vi "FL_Calculate_phi_theta_etc_for_saving.vi"(3 "Mouse face dir. swap":bool, 4 "Input cluster of data":T1) -> (1 "Output data cluster":T2)   [LabVIEW 2016]
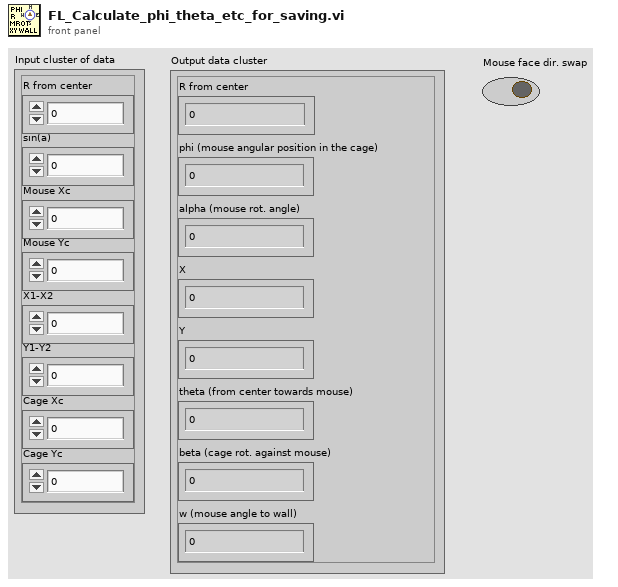
[diagram p1: front panel]
types:
  T1 = cluster{"R from center":dbl, "sin(a)":dbl, "Mouse Xc":dbl, "Mouse Yc":dbl, "X1-X2":dbl, "Y1-Y2":dbl, "Cage Xc":dbl, "Cage Yc":dbl}
  T2 = cluster{"R from center":dbl, "phi (mouse angular position in the cage)":dbl, "alpha (mouse rot. angle)":sgl, "X":dbl, "Y":dbl, "theta (from center towards mouse)":dbl, "beta (cage rot. against mouse)":sgl, "w (mouse angle to wall)":dbl}
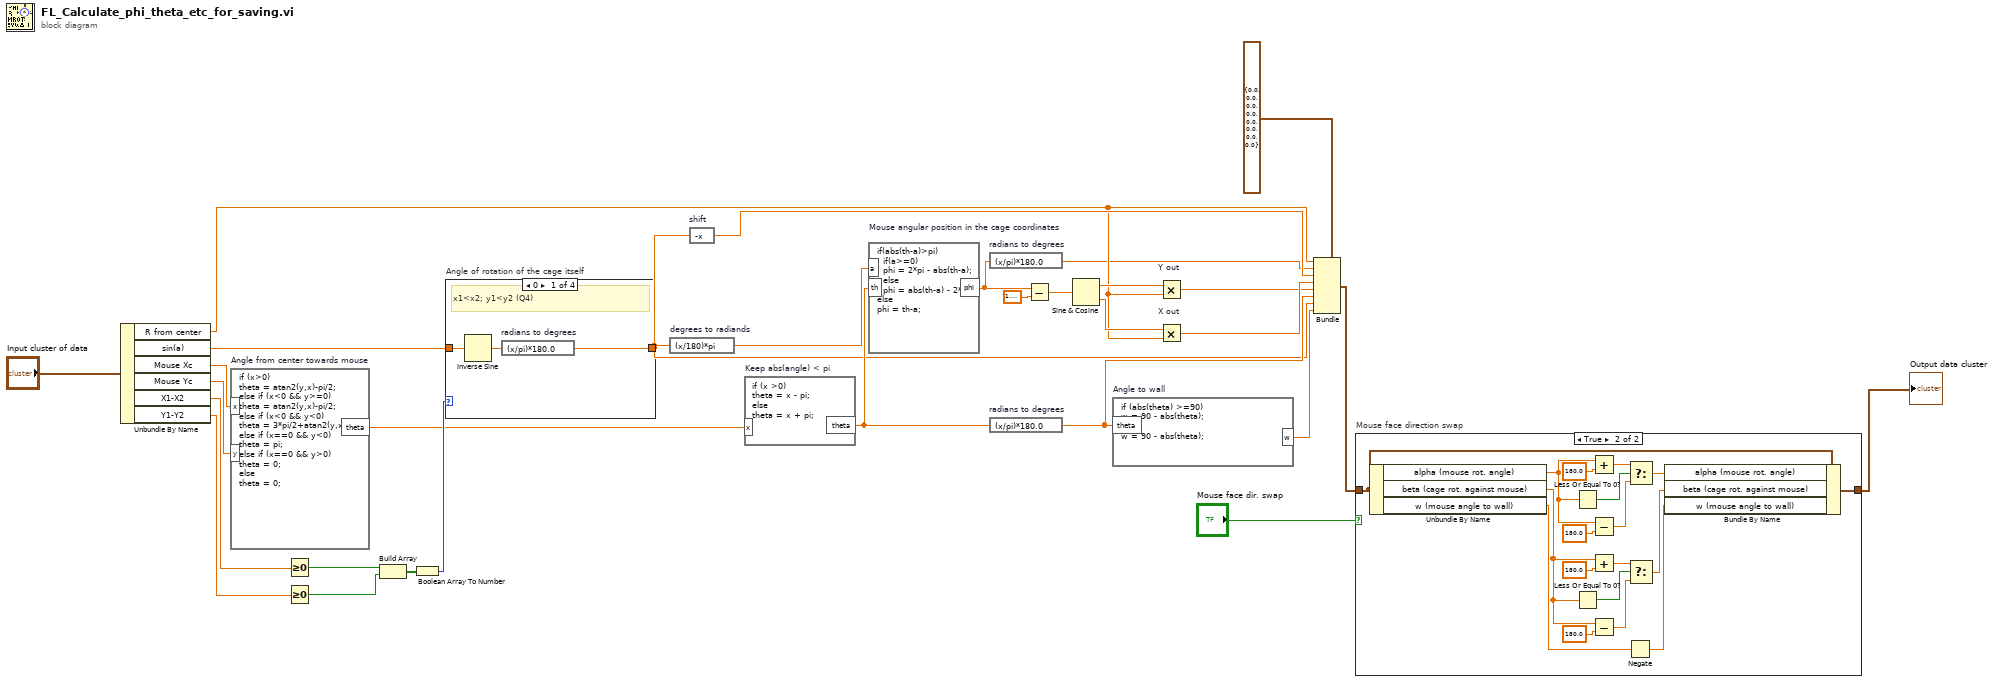
[diagram p0: block diagram]
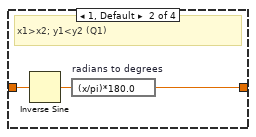
[diagram p3: hidden frame]
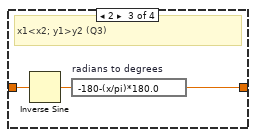
[diagram p4: hidden frame]
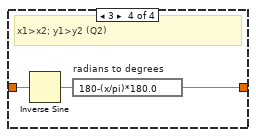
[diagram p5: hidden frame]
diagram:
  n1 = Unbundle By Name("Input cluster of data") -> ("R from center"=w6:dbl, "sin(a)"=w12:dbl, "Mouse Xc"=w11:dbl, "Mouse Yc"=w10:dbl, "X1-X2"=w9:dbl, "Y1-Y2"=w8:dbl)
  n2 = formula code="if (x>0)\ntheta = atan2(y,x)-pi/2;\nelse if (x<0 && y>=0)\ntheta = atan2(y,x)-pi/2;\nelse if (x<0 && y<0)\ntheta = 3*pi/2+atan2(y,x);\nelse if (x==0 && y<0)\ntheta = pi;\nelse if (x==0 && y>0)\ntheta = 0;\nelse\ntheta = 0;" "Angle from center towards mouse"("x"=w11, "y"=w10) -> ("theta"=w26:dbl)
  n3 = Greater Or Equal To 0?(x=w9) -> (x >= 0?=w30:bool)
  n4 = Greater Or Equal To 0?(x=w8) -> (x >= 0?=w29:bool)
  n5 = Build Array(w30, w29) -> (w28:bool[])
  n6 = Boolean Array To Number(Boolean array=w28) -> (number=w27:u32)
  n7 = case "Angle of rotation of the cage itself" shown="0" w27 {
    tunnel: w12 -> [w32 w35 w38 w41]
    tunnel: [w31 w34 w37 w40] -> w15
    frame 0 {
      # "x1<x2; y1<y2 (Q4)"
      n8 = Inverse Sine(1:w32) -> (0:w33:dbl)
      n9 = expression code="(x/pi)*180.0" "radians to degrees"(w33) -> (w31:dbl)
    }
    frame 1, Default {
      # "x1>x2; y1<y2 (Q1)"
      n10 = Inverse Sine(1:w35) -> (0:w36:dbl)
      n11 = expression code="(x/pi)*180.0" "radians to degrees"(w36) -> (w34:dbl)
    }
    frame 2 {
      # "x1<x2; y1>y2 (Q3)"
      n12 = Inverse Sine(1:w38) -> (0:w39:dbl)
      n13 = expression code="-180-(x/pi)*180.0" "radians to degrees"(w39) -> (w37:dbl)
    }
    frame 3 {
      # "x1>x2; y1>y2 (Q2)"
      n14 = Inverse Sine(1:w41) -> (0:w42:dbl)
      n15 = expression code="180-(x/pi)*180.0" "radians to degrees"(w42) -> (w40:dbl)
    }
  }
  n16 = expression code="(x/180)*pi" "degrees to radiands"(w15) -> (w22:dbl)
  n17 = expression code="-x" "shift"(w15) -> (w7:dbl)
  n18 = formula code="if (x >0)\ntheta = x - pi;\nelse\ntheta = x + pi;" "Keep abs(angle) < pi"("x"=w26) -> ("theta"=w23:dbl)
  n19 = formula code="if(abs(th-a)>pi)\n  if(a>=0)\n  phi = 2*pi - abs(th-a);\n  else\n  phi = abs(th-a) - 2*pi;\nelse\nphi = th-a;" "Mouse angular position in the cage coordinates"("th"=w23, "a"=w22) -> ("phi"=w20:dbl)
  n20 = expression code="(x/pi)*180.0" "radians to degrees"(w20) -> (w5:dbl)
  n21 = expression code="(x/pi)*180.0" "radians to degrees"(w23) -> (w16:dbl)
  n22 = Subtract(x=w20, y=1.5707963267948966) -> (x-y=w21:dbl)
  n23 = Sine & Cosine(0:w21) -> (1:w24:dbl, 2:w25:dbl)
  n24 = formula code="if (abs(theta) >=90)\nw = 90 - abs(theta);\nelse\nw = 90 - abs(theta);" "Angle to wall"("theta"=w16) -> ("w"=w14:dbl)
  n25 = Multiply "Y out"(x=w24, y=w6) -> (x*y=w17:dbl)
  n26 = Multiply "X out"(x=w25, y=w6) -> (x*y=w18:dbl)
  n27 = Bundle(cluster=T2 {"R from center"=0.0, "phi (mouse angular position in the cage)"=0.0, "alpha (mouse rot. angle)"=0.0, "X"=0.0, "Y"=0.0, "theta (from center towards mouse)"=0.0, "beta (cage rot. against mouse)"=0.0, "w (mouse angle to wall)"=0.0} ("Output data cluster 2"), "R from center"=w6, "phi (mouse angular position in the cage)"=w5, "alpha (mouse rot. angle)"=w7, "X"=w18, "Y"=w17, "theta (from center towards mouse)"=w16, "beta (cage rot. against mouse)"=w15, "w (mouse angle to wall)"=w14) -> (w2:T2)
  n28 = case "Mouse face direction swap" shown="True" "Mouse face dir. swap" {
    tunnel: [w43 w55] -> w1
    tunnel: w2 -> [w43 w56]
    frame False {
    }
    frame True {
      n29 = Unbundle By Name(w56) -> ("alpha (mouse rot. angle)"=w54:sgl, "beta (cage rot. against mouse)"=w47:sgl, "w (mouse angle to wall)"=w45:dbl)
      n30 = Less Or Equal To 0?(x=w54) -> (x <= 0?=w61:bool)
      n31 = Less Or Equal To 0?(x=w47) -> (x <= 0?=w48:bool)
      n32 = Add(x=w54, y=sgl 180.0) -> (x+y=w58:sgl)
      n33 = Subtract(x=w54, y=sgl 180.0) -> (x-y=w60:sgl)
      n34 = Add(x=w47, y=sgl 180.0) -> (x+y=w51:sgl)
      n35 = Subtract(x=w47, y=sgl 180.0) -> (x-y=w49:sgl)
      n36 = Negate(x=w45) -> (-x=w44:dbl)
      n37 = Select(t=w58, s=w61, f=w60) -> (s? t:f=w53:sgl)
      n38 = Select(t=w51, s=w48, f=w49) -> (s? t:f=w46:sgl)
      n39 = Bundle By Name(cluster=w56, "alpha (mouse rot. angle)"=w53, "beta (cage rot. against mouse)"=w46, "w (mouse angle to wall)"=w44) -> (w55:T2)
    }
  }
  "Output data cluster" <- w1
